vi "Execute Subscription Policy.vi"(9 "Publish Time":timestamp, 10 "New Topic Value":variant, 11 "Subscription Policy":T1) -> (0 "error out (Unsubscribe?)":errorcluster, 3 "Subscription Policy Out":T1)   [LabVIEW 2017, in "IMediator.lvlib" / "ISubscriptionPolicy.lvclass"]
doc: "This method decides whether or not to send or otherwise handle the new data value. The policy is set and maintained by the subscriber. The Topic Actor knows no policy details, it just passes the new value in. If there is a failure inside this method, the Topic Actor must assume the listener is no longer valid (dead/unrecoverable) and should delete it from the Subscriber list.\n\n<License>\nCopyright © 2017 Composed Systems, LLC | All rights reserved\nwww.composed.io\n\nAuthor: Ethan Stern <ethan.stern@composed.io>\n\nThis software is provided \"AS IS\" WITHOUT WARRANTIES, either express or implied, AND IS FOR EDUCATIONAL PURPOSES ONLY.\n</License>"
uses:
  ISubscriptionPolicy.lvclass
  ISubscriptionPolicy Reference.ctl
  ISubscriptionPolicy.lvclass/ISubscriptionPolicy.ctl
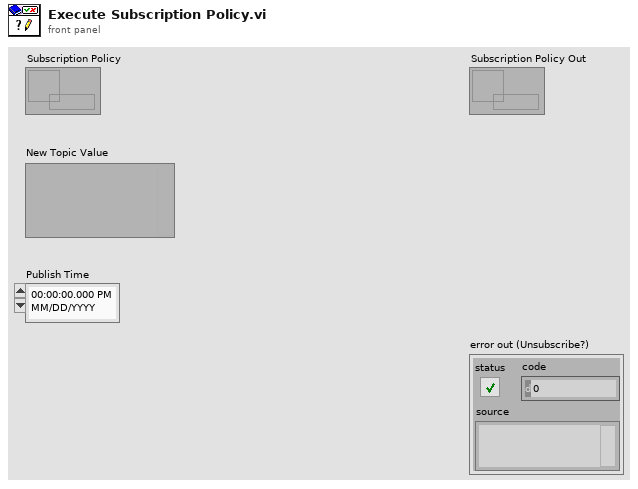
[diagram p1: front panel]
types:
  T1 = typedef "IMediator.lvlib/ISubscriptionPolicy.lvclass/ISubscriptionPolicy Reference.ctl" = refnum<data-value>
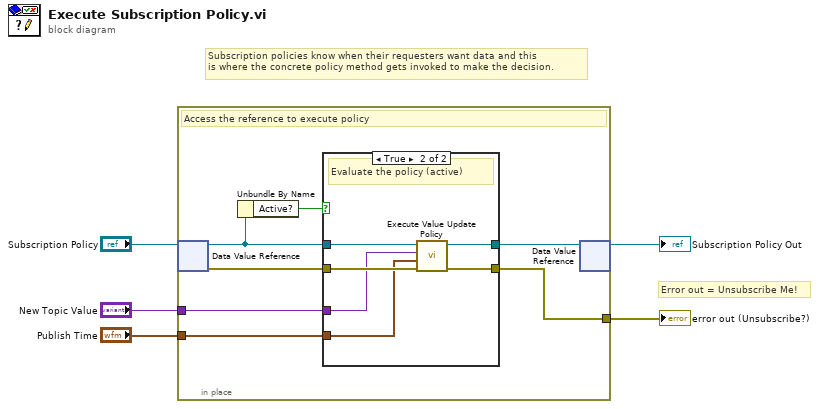
[diagram p0: block diagram]
diagram:
  # "Error out = Unsubscribe Me!"
  # "Subscription policies know when their requesters want data and this\nis where the concrete policy method gets invoked to make the decision."
  n1 = in-place {
    in-place-border: "New Topic Value" -> [w10]
    in-place-border: "Publish Time" -> [w9]
    in-place-border: [w8] -> w1
    # "Access the reference to execute policy"
    n2 = in-place-dvr #1("Subscription Policy") -> (w7:refnum<class "ISubscriptionPolicy.lvclass">, w11:errorcluster)
    n3 = Unbundle By Name(w7) -> ("Active?"=w6:bool)
    n4 = case shown="True" w6 {
      tunnel: w7 -> [w14 w20]
      tunnel: [w14 w19] -> w12
      tunnel: w11 -> [w13 w18]
      tunnel: w10 -> [_ w17]
      tunnel: w9 -> [_ w16]
      tunnel: [w13 w15] -> w8
      frame False {
        # "Skip evaluation (not active)"
      }
      frame True {
        # "Evaluate the policy (active)"
        n5 = call-dynamic "Execute Value Update Policy.vi"("error in (no error)"=w18, "Publish Time"=w16, "New Topic Value"=w17, "ISubscriptionPolicy In"=w20) -> ("error out"=w15:errorcluster, "ISubscriptionPolicy Out"=w19:refnum<class "ISubscriptionPolicy.lvclass">)  [unwired: 6 in]
      }
    }
    n6 = in-place-dvr #1(w12) -> (→"Subscription Policy Out":T1)  [unwired: 1 out]
  }
  "error out (Unsubscribe?)" <- w1
